vi "setRotAng.vi"(8 "error in (no error)":errorcluster, 10 "Rotation Angle in Deg":dbl, 11 "CamRot in":refnum<class "CamRot.lvclass">) -> (0 "error out":errorcluster, 3 "CamRot out":refnum<class "CamRot.lvclass">)   [LabVIEW 2016, in "CamRot.lvclass"]
doc: "Set the rotation angle in degree."
uses:
  CamRot.lvclass
  CamRot.lvclass/CamRot.ctl
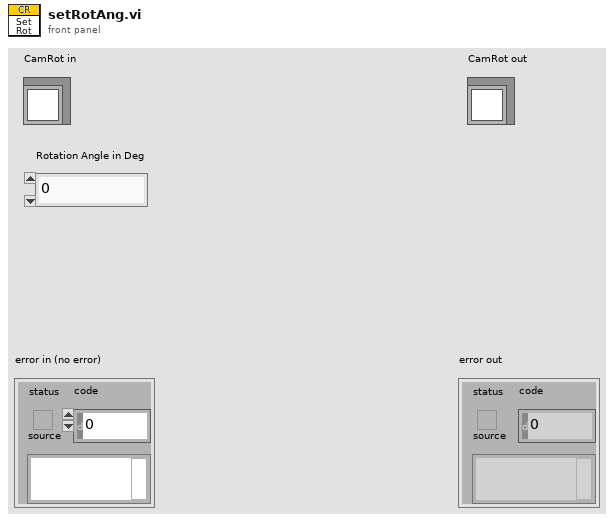
[diagram p1: front panel]
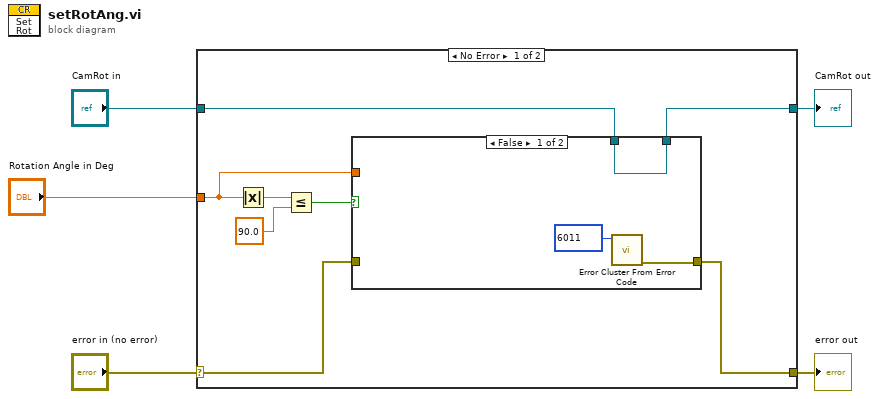
[diagram p0: block diagram]
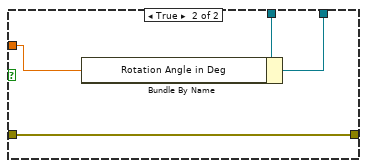
[diagram p2: hidden frame]
diagram:
  n1 = case shown="No Error" "error in (no error)" {
    selector: "error in (no error)" -> [w7 w22]
    tunnel: [w6 w22] -> w4
    tunnel: [w12 w21] -> w2
    tunnel: "CamRot in" -> [w13 w21]
    tunnel: "Rotation Angle in Deg" -> [w8 _]
    frame No Error {
      n2 = Absolute Value(x=w8) -> (abs(x)=w11:dbl)
      n3 = Less Or Equal?(x=w11, y=90.0) -> (x <= y?=w9:bool)
      n4 = case shown="False" w9 {
        tunnel: w13 -> [w14 w20]
        tunnel: [w14 w19] -> w12
        tunnel: w8 -> [_ w18]
        tunnel: w7 -> [_ w17]
        tunnel: [w16 w17] -> w6
        frame False {
          n5 = call <vilib>:"Error Cluster From Error Code.vi"("error code (0)"=6011) -> ("error out"=w16:errorcluster)  [unwired: 8 in]
        }
        frame True {
          n6 = Bundle By Name(cluster=w20, "Rotation Angle in Deg"=w18) -> (w19:refnum<class "CamRot.lvclass">)
        }
      }
    }
    frame Error {
    }
  }
  "error out" <- w4
  "CamRot out" <- w2
